vi "Read Line Rate - With Two Methods - Returns Total Value.vi"() -> ()   [LabVIEW 2017, in "Cobertura.Tests.lvlib" / "Coverage.lvlib"]
uses:
  Coverage.lvlib
  Cobertura/Coverage/Coverage.lvclass/Coverage.ctl
  Cobertura/Coverage/Read Line Rate.vi
  <vilib>/PNR/Transparent Assertions/Transparent Assertions/Transparent Assertions.lvlib
  Cobertura/Package/Package.lvclass
  Cobertura/Class/Class.lvclass
  Cobertura/Method/Method.lvclass
  Cobertura/Coverage/Coverage.lvclass
panel:
  out "error out":errorcluster
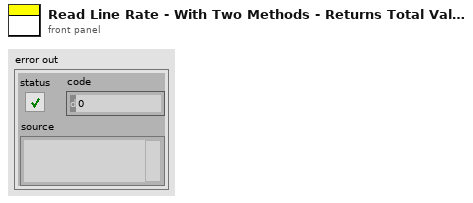
[diagram p1: front panel]
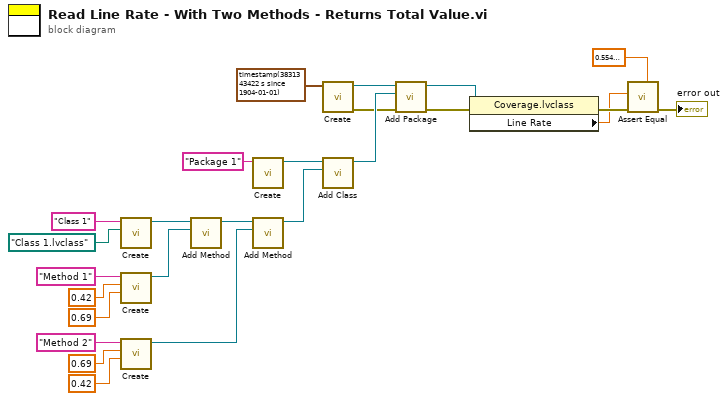
[diagram p0: block diagram]
diagram:
  n1 = call "Create.vi"("Filename"=path "Class 1.lvclass", "Name"="Class 1") -> ("Class"=w22:refnum<class "Class.lvclass">)  [unwired: 8 in, 1 out]
  n2 = call "Create.vi"("Branch Rate"=0.69, "Line Rate"=0.42, "Name"="Method 1") -> ("Method"=w18:refnum<class "Method.lvclass">)  [unwired: 7 in, 1 out]
  n3 = call "Create.vi"("Branch Rate"=0.42, "Line Rate"=0.69, "Name"="Method 2") -> ("Method"=w13:refnum<class "Method.lvclass">)  [unwired: 7 in, 1 out]
  n4 = call "Add Method.vi"("Method"=w18, "Class in"=w22) -> ("Class out"=w14:refnum<class "Class.lvclass">)  [unwired: 8 in, 1 out]
  n5 = call "Create.vi"("Name"="Package 1") -> ("Package"=w8:refnum<class "Package.lvclass">)  [unwired: 9 in, 1 out]
  n6 = call "Add Method.vi"("Method"=w13, "Class in"=w14) -> ("Class out"=w10:refnum<class "Class.lvclass">)  [unwired: 8 in, 1 out]
  n7 = call "Create.vi"("Timestamp"=timestamp(3831343422.3303647 s since 1904-01-01)) -> ("error out"=w4:errorcluster, "Coverage"=w7:refnum<class "Coverage.lvclass">)  [unwired: 9 in]
  n8 = call "Add Class.vi"("Class"=w10, "Package in"=w8) -> ("Package out"=w5:refnum<class "Package.lvclass">)  [unwired: 8 in, 1 out]
  n9 = call "Add Package.vi"("error in (no error)"=w4, "Package"=w5, "Coverage in"=w7) -> ("error out"=w6:errorcluster, "Coverage out"=w3:refnum<class "Coverage.lvclass">)  [unwired: 7 in]
  n10 = property class="Coverage.lvclass"(reference=w3, error in=w6) -> (error out=w24:errorcluster, "Line Rate"=w12:dbl)  [unwired: 1 out]
  n11 = call <vilib>:"Assert Equal.vi"("Expected"=0.5549999999999999 ("Branch Rate"), "error in (no error)"=w24, "Actual"=w12) -> ("error out"=→"error out":errorcluster)  [unwired: 8 in]
